vi "QCA Pick Baseline.vi"(1 "QMeter":string, 2 "Current Baseline":i32) -> (0 "New Baseline":i32)   [LabVIEW 2009]
doc: "This VI is called by the QCA. Its purpose is to present the user with a range of choices for what baseline to use. The user can pick from existing baselines for the current Q Meter, or can opt to take a new baseline."
panel:
  in  "No Baseline":bool
  in  "Cancel":bool
  in  "New Baseline":bool
  in  "Choose Baseline":bool
  out "Raw Signal of Highlighted Baseline":dbl[](graph)
  in  "To choose an existing baseline, select from this list":i32(listbox)
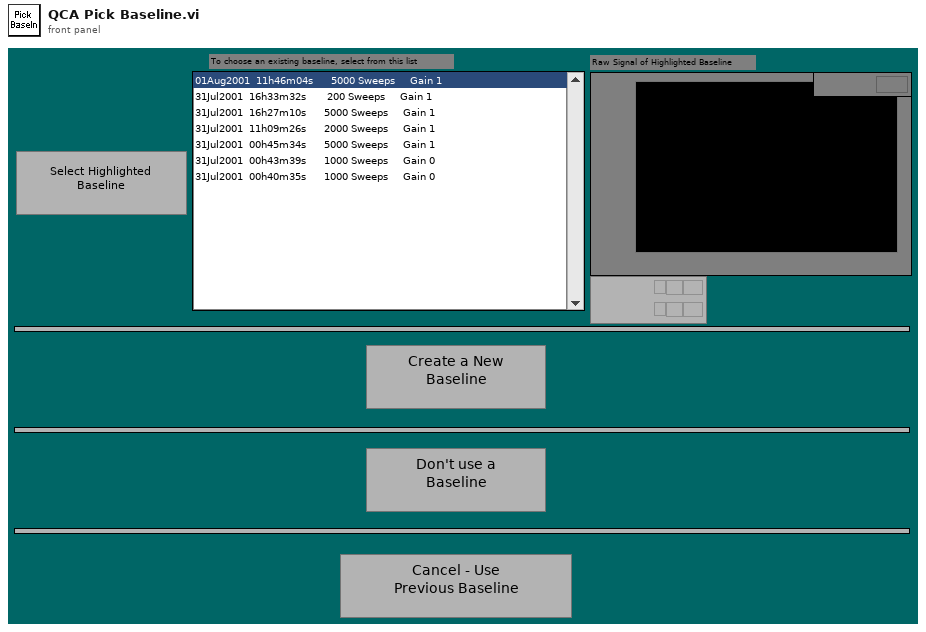
[diagram p1: front panel]
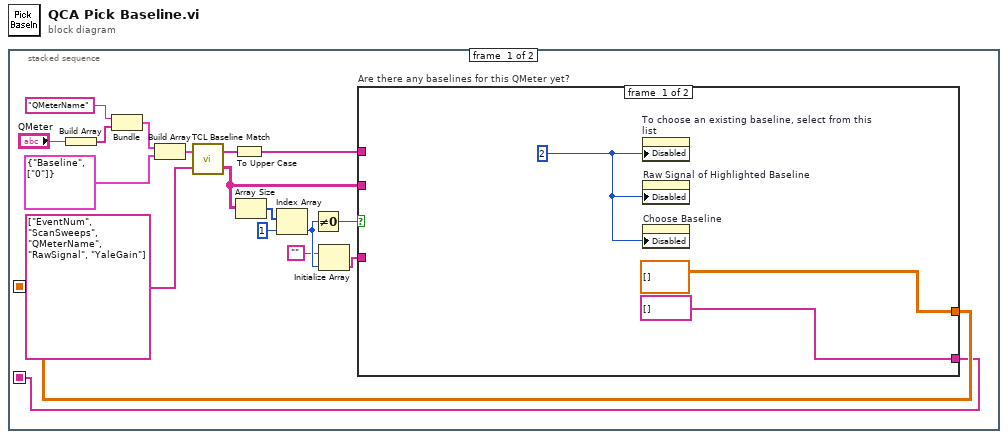
[diagram p0: block diagram]
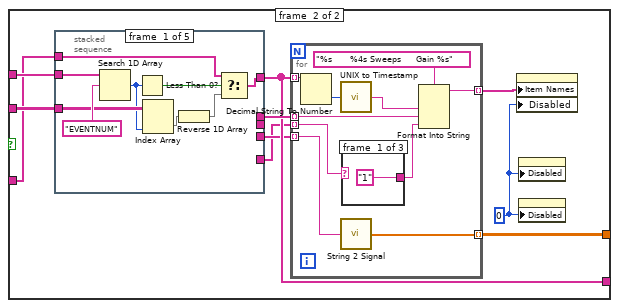
[diagram p2: hidden frame]
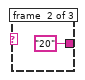
[diagram p3: hidden frame]
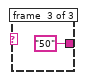
[diagram p4: hidden frame]
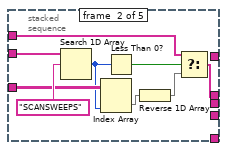
[diagram p5: hidden frame]
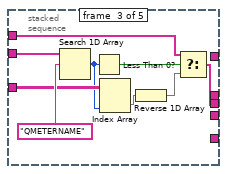
[diagram p6: hidden frame]
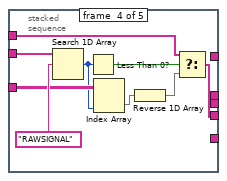
[diagram p7: hidden frame]
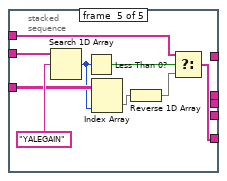
[diagram p8: hidden frame]
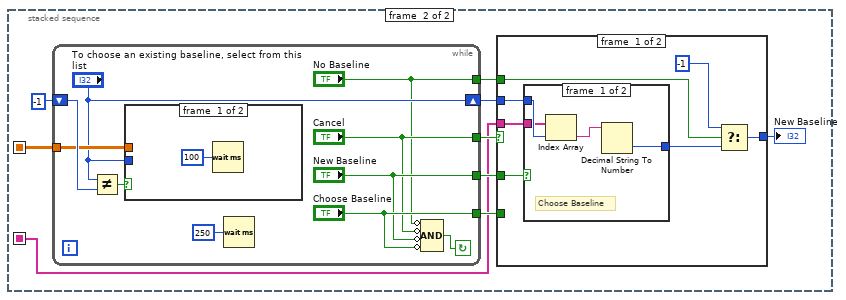
[diagram p9: hidden frame]
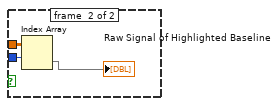
[diagram p10: hidden frame]
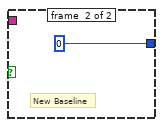
[diagram p11: hidden frame]
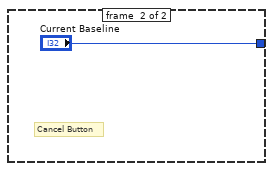
[diagram p12: hidden frame]
diagram:
  n1 = stacked-sequence {
    seq-local: [w7 _] -> [_ w97]
    seq-local: [w6 _] -> [_ w92]
    frame #0 {
      n2 = Build Array("QMeter") -> (w16:string[])
      n3 = Bundle("QMeterName", w16) -> (w15:cluster{string, string[]})  [unwired: 1 in]
      n4 = Build Array(w15, cluster{string, string[]} {"Baseline", ["0"]}) -> (w13:cluster{string, string[]}[])
      n5 = call "TCL Baseline Match.vi"("Fragments Desired"=string[] ["EventNum", "ScanSweeps", "QMeterName", "RawSignal", "YaleGain"], "Fragments to Match"=w13) -> ("Event Data"=w9:string[][], "Fragments Returned"=w10:string[])
      n6 = To Upper Case(1:w10) -> (0:w8:string[])
      n7 = Array Size(array=w9) -> (size(s)=w5:i32[])
      n8 = Index Array(array=w5, index=1) -> (element=w3:i32)
      n9 = Not Equal To 0?(x=w3) -> (x != 0?=w11:bool)
      n10 = Initialize Array("", w3) -> (w1:string[])
      n11 = case "Are there any baselines for this QMeter yet?" shown="True" w11 {
        tunnel: w8 -> [_ w31]
        tunnel: w9 -> [_ w30]
        tunnel: [dbl[][] [] ("Raw Signal") w24] -> w7
        tunnel: [string[] [] ("Event Data") w26] -> w6
        tunnel: w1 -> [_ w27]
        frame #0 {
          w21 = 2
          n12 = property on="To choose an existing baseline, select from this list" class="ListBox (strict)"("Disabled"=w21) -> ()  [unwired: 2 in, 2 out]
          n13 = property on="Raw Signal of Highlighted Baseline" class="WaveformGraph (strict)"("Disabled"=w21) -> ()  [unwired: 2 in, 2 out]
          n14 = property on="Choose Baseline" class="Boolean"("Disabled"=w21) -> ()  [unwired: 2 in, 2 out]
        }
        frame #1 {
          w28 = u8 0
          n15 = stacked-sequence {
            tunnel: w30 -> [w52 w61 w70 w79 w88]
            tunnel: w31 -> [w51 w60 w69 w78 w87]
            tunnel: [w46 _ _ _ _] -> w26
            tunnel: [_ w55 _ _ _] -> w29
            tunnel: [_ _ w64 _ _] -> _
            tunnel: [_ _ _ w73 _] -> w25
            tunnel: w27 -> [w50 w59 w68 w77 w86]
            tunnel: [_ _ _ _ w82] -> w22
            frame #0 {
              n16 = Search 1D Array(1D array=w51, element="EVENTNUM") -> (index of element=w47:i32)  [unwired: 1 in]
              n17 = Less Than 0?(x=w47) -> (x < 0?=w48:bool)
              n18 = Index Array(array=w52, index (col)=w47) -> (element=w49:string[])  [unwired: 1 in]
              n19 = Reverse 1D Array(array=w49) -> (reversed array=w45:string[])
              n20 = Select(t=w50, s=w48, f=w45) -> (s? t:f=w46:string[])
            }
            frame #1 {
              n21 = Search 1D Array(1D array=w60, element="SCANSWEEPS") -> (index of element=w56:i32)  [unwired: 1 in]
              n22 = Index Array(array=w61, index (col)=w56) -> (element=w58:string[])  [unwired: 1 in]
              n23 = Less Than 0?(x=w56) -> (x < 0?=w57:bool)
              n24 = Reverse 1D Array(array=w58) -> (reversed array=w54:string[])
              n25 = Select(t=w59, s=w57, f=w54) -> (s? t:f=w55:string[])
            }
            frame #2 {
              n26 = Search 1D Array(1D array=w69, element="QMETERNAME") -> (index of element=w65:i32)  [unwired: 1 in]
              n27 = Less Than 0?(x=w65) -> (x < 0?=w66:bool)
              n28 = Index Array(array=w70, index (col)=w65) -> (element=w67:string[])  [unwired: 1 in]
              n29 = Reverse 1D Array(array=w67) -> (reversed array=w63:string[])
              n30 = Select(t=w68, s=w66, f=w63) -> (s? t:f=w64:string[])
            }
            frame #3 {
              n31 = Search 1D Array(1D array=w78, element="RAWSIGNAL") -> (index of element=w74:i32)  [unwired: 1 in]
              n32 = Less Than 0?(x=w74) -> (x < 0?=w75:bool)
              n33 = Index Array(array=w79, index (col)=w74) -> (element=w76:string[])  [unwired: 1 in]
              n34 = Reverse 1D Array(array=w76) -> (reversed array=w72:string[])
              n35 = Select(t=w77, s=w75, f=w72) -> (s? t:f=w73:string[])
            }
            frame #4 {
              n36 = Search 1D Array(1D array=w87, element="YALEGAIN") -> (index of element=w83:i32)  [unwired: 1 in]
              n37 = Less Than 0?(x=w83) -> (x < 0?=w84:bool)
              n38 = Index Array(array=w88, index (col)=w83) -> (element=w85:string[])  [unwired: 1 in]
              n39 = Reverse 1D Array(array=w85) -> (reversed array=w81:string[])
              n40 = Select(t=w86, s=w84, f=w81) -> (s? t:f=w82:string[])
            }
          }
          n41 = for {
            tunnel: w26 -> [w41] mode=indexing
            tunnel: w29 -> [w34] mode=indexing
            tunnel: w22 -> [w33] mode=indexing
            tunnel: [w37] -> w23 mode=indexing
            tunnel: w25 -> [w36] mode=indexing
            tunnel: [w35] -> w24 mode=indexing
            n42 = Decimal String To Number(string=w41) -> (number=w40:i32)  [unwired: 2 in, 1 out]
            n43 = call "UNIX to Timestamp.vi"("Seconds"=w40) -> ("Timestamp String"=w39:string)
            n44 = call "String 2 Signal.vi"("String"=w36) -> ("Signal"=w35:dbl[])
            n45 = case shown="\"0\", Default" w33 {
              tunnel: ["1" "20" "50"] -> w32
              frame #0 {
              }
              frame #1 {
              }
              frame #2 {
              }
            }
            n46 = Format Into String(format string="%s      %4s Sweeps     Gain %s", w39, w34, w32) -> (resulting string=w37:string)  [unwired: 2 in, 1 out]
          }
          n47 = property on="To choose an existing baseline, select from this list" class="ListBox (strict)"("Item Names"=w23, "Disabled"=w28) -> ()  [unwired: 2 in, 2 out]
          n48 = property on="Raw Signal of Highlighted Baseline" class="WaveformGraph (strict)"("Disabled"=w28) -> ()  [unwired: 2 in, 2 out]
          n49 = property on="Choose Baseline" class="Boolean"("Disabled"=w28) -> ()  [unwired: 2 in, 2 out]
        }
      }
    }
    frame #1 {
      n50 = while {
        tunnel: ["No Baseline"] -> w90
        tunnel: ["Cancel"] -> w96
        tunnel: ["New Baseline"] -> w95
        tunnel: ["Choose Baseline"] -> w94
        tunnel: w97 -> [w106]
        shift-left: -1 -> [w108]
        shift-right: ["To choose an existing baseline, select from this list"] -> w93
        stop <- w104 continue-if-true
        n51 = Not Equal?(x="To choose an existing baseline, select from this list", y=w108) -> (x != y?=w107:bool)
        n52 = case shown="True" w107 {
          tunnel: w106 -> [_ w111]
          tunnel: "To choose an existing baseline, select from this list" -> [_ w112]
          frame #0 {
            n53 = Wait (ms)(milliseconds to wait=u32 100) -> ()  [unwired: 1 out]
          }
          frame #1 {
            n54 = Index Array(array=w111, index (row)=w112) -> (element=→"Raw Signal of Highlighted Baseline":dbl[])  [unwired: 1 in]
          }
        }
        n55 = Wait (ms)(milliseconds to wait=u32 250) -> ()  [unwired: 1 out]
        n56 = Compound Arithmetic op=AND(invert "No Baseline", invert "Cancel", invert "New Baseline", invert "Choose Baseline") -> (w104:bool)
      }
      n57 = case shown="False" w96 {
        tunnel: w95 -> [w117 _]
        tunnel: w94 -> [_ _]
        tunnel: [w116 "Current Baseline"] -> w91
        tunnel: w93 -> [w119 _]
        tunnel: w92 -> [w118 _]
        tunnel: w90 -> [w114 _]
        frame #0 {
          n58 = case shown="False" w117 {
            tunnel: [w120 0] -> w115
            tunnel: w119 -> [w123 _]
            tunnel: w118 -> [w122 _]
            frame #0 {
              # "Choose Baseline"
              n59 = Index Array(array=w122, index=w123) -> (element=w121:string)
              n60 = Decimal String To Number(string=w121) -> (number=w120:i32)  [unwired: 2 in, 1 out]
            }
            frame #1 {
              # "New Baseline"
            }
          }
          n61 = Select(t=-1, s=w114, f=w115) -> (s? t:f=w116:i32)
        }
        frame #1 {
          # "Cancel Button"
        }
      }
      "New Baseline" <- w91
    }
  }
